vi "Start.vi"(6 "Teller":T1 {"AbsoluteTime" format="%<%x %.3X>T"}, 8 "Error in":errorcluster, 11 "Base Actor in":refnum<class "Base Actor.lvclass">) -> (0 "Error out":errorcluster, 3 "Base Actor out":refnum<class "Base Actor.lvclass">)   [LabVIEW 2020, in "jettl.lvlib" / "BaseActor.lvlib" / "Base Actor.lvclass"]
doc: "jettl 6.14.1.98\nNathan Davis - Nathan Davis\nCopyright (c) 2026, Nathan Davis\nMIT"
uses:
  Base Actor.lvclass
  Base Actor.lvclass/Base Actor.ctl
  ActorRelation.ctl
  jettl.lvlib
  MessageMetadata.ctl
  ActorLifetime.ctl
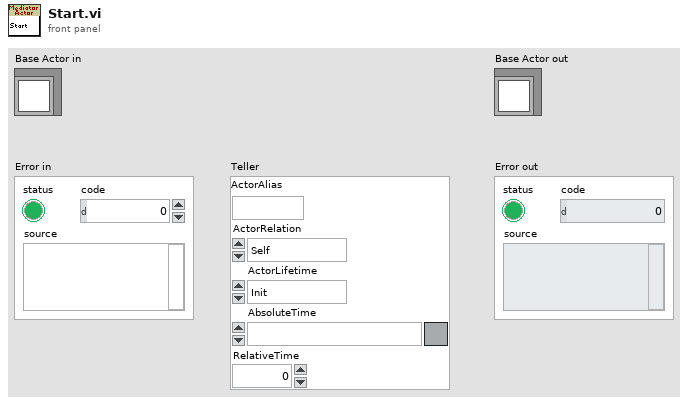
[diagram p1: front panel]
types:
  T1 = typedef "jettl.lvlib/MessageMetadata.ctl" = cluster{"ActorAlias":string, "ActorRelation":T2, "ActorLifetime":T3, "AbsoluteTime":timestamp, "RelativeTime":dbl}
  T2 = typedef "jettl.lvlib/ActorRelation.ctl" = enum16{"Self", "Mediator", "Component"}
  T3 = typedef "jettl.lvlib/ActorLifetime.ctl" = enum16{"Init", "Spawn", "Setup", "Teardown Before Running", "Running", "Stop Called", "Stopping With Children", "Stopping Without Children", "Teardown After Running", "Stopped"}
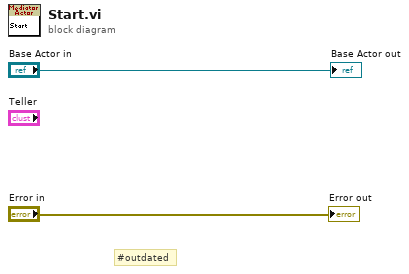
[diagram p0: block diagram]
diagram:
  # "#outdated"
  "Base Actor out" <- "Base Actor in"
  "Error out" <- "Error in"
